vi "校准记录.vi"(8 "error in (no error)":errorcluster, 9 "曲线模型":T1={"标液浓度1"=0.0, "测量吸光度1"=0.0, "样品1启用"=FALSE, "标液浓度2"=0.0, "测量吸光度2"=0.0, "样品2启用"=FALSE, "标液浓度3"=0.0, "测量吸光度3"=0.0, "样品3启用"=FALSE, "标液浓度4"=0.0, "测量吸光度4"=0.0, "样品4启用"=FALSE, "标液浓度5"=0.0, "测量吸光度5"=0.0, "样品5启用"=FALSE, "模型"=enum."线性", "精度"=4.0, "XY图"=[], "拟合公式"="", "r^2"=0.0, "标样一校准时间"=timestamp(0 s since 1904-01-01), "标样二校准时间"=timestamp(0 s since 1904-01-01), "标样三校准时间"=timestamp(0 s since 1904-01-01), "标样四校准时间"=timestamp(0 s since 1904-01-01), "标样五校准时间"=timestamp(0 s since 1904-01-01), "二次方程"={"c"=0.0, "x"=0.0, "x^2"=0.0}, "标定时间"=timestamp(0 s since 1904-01-01), "拟合公式 2"="", "r^2 2"=0.0} {"r^2 2" format="%.7f"; "标定时间" format="%<%m/%d/%y %H:%M:%S>T"; "标样五校准时间" format="%<%m/%d/%y %H:%M:%S>T"; "标样四校准时间" format="%<%m/%d/%y %H:%M:%S>T"; "标样三校准时间" format="%<%m/%d/%y %H:%M:%S>T"; "标样二校准时间" format="%<%m/%d/%y %H:%M:%S>T"; "标样一校准时间" format="%<%m/%d/%y %H:%M:%S>T"; "r^2" format="%.7f"; "测量吸光度5" format="%#.6f"; "测量吸光度4" format="%#.6f"; "测量吸光度3" format="%#.6f"; "测量吸光度2" format="%#.6f"; "测量吸光度1" format="%#.6f"}, 10 "量程":enum16{"低量程", "高量程"}(ring), 11 "校准参数":u16(ring) items=["总氮"=2, "总磷"=1]) -> (0 "error out":errorcluster)   [LabVIEW 2016, in "斯坦道CODMn新电路板.lvlib"]
uses:
  <vilib>/addons/database/Auxilliary.llb/DB Tools Column Info.ctl
  <vilib>/addons/database/Auxilliary.llb/DB Tools DataTypes.ctl
  <vilib>/addons/database/NI_Database_API.lvlib
  <vilib>/Utility/VariantDataType/VariantType.lvlib
panel:
  out "结果字符串":string
  in  "data in":T2
  # "校准时间"
  # "标液浓度"
  # "吸光值显示"
  # "标液一"
  # "标液二"
  # "标液三"
  # "零点"
  # "跨度"
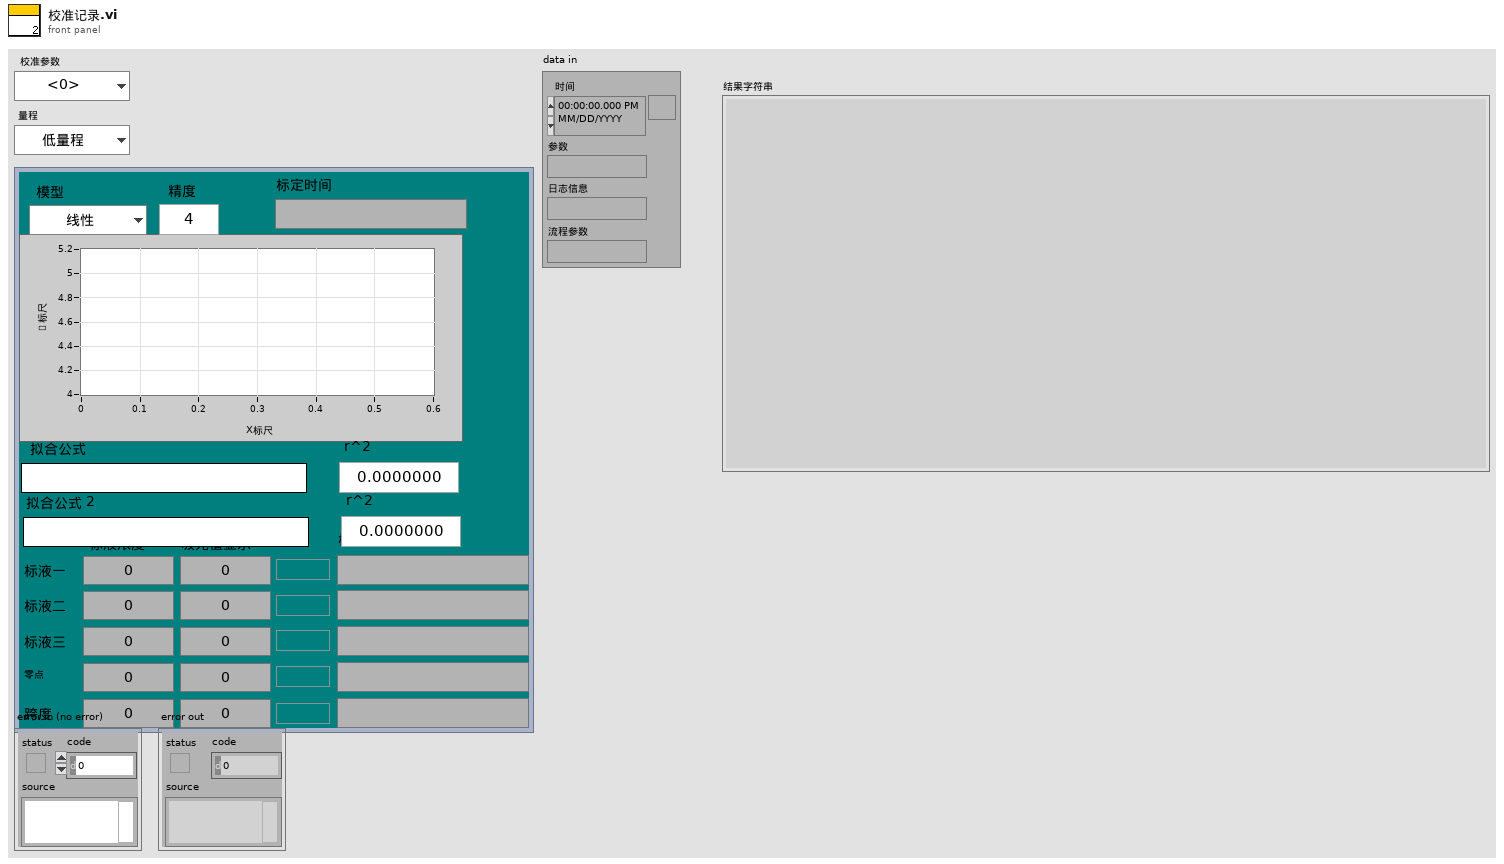
[diagram p1: front panel]
types:
  T1 = cluster{"标液浓度1":dbl, "测量吸光度1":dbl, "样品1启用":bool, "标液浓度2":dbl, "测量吸光度2":dbl, "样品2启用":bool, "标液浓度3":dbl, "测量吸光度3":dbl, "样品3启用":bool, "标液浓度4":dbl, "测量吸光度4":dbl, "样品4启用":bool, "标液浓度5":dbl, "测量吸光度5":dbl, "样品5启用":bool, "模型":enum32{"线性", "多项式", "折线"}, "精度":dbl, "XY图":cluster{"X Values":dbl[], "Y Values":dbl[]}[], "拟合公式":string, "r^2":dbl, "标样一校准时间":timestamp, "标样二校准时间":timestamp, "标样三校准时间":timestamp, "标样四校准时间":timestamp, "标样五校准时间":timestamp, "二次方程":cluster{"c":dbl, "x":dbl, "x^2":dbl}, "标定时间":timestamp, "拟合公式 2":string, "r^2 2":dbl}
  T2 = cluster{"时间":timestamp, "参数":string, "日志信息":string, "流程参数":string}
  T3 = typedef "NI_Database_API.lvlib/DB Tools Column Info.ctl" = cluster{"column name":string, "data type":T4, "size":i32, "allow null?":bool}
  T4 = typedef "NI_Database_API.lvlib/DB Tools DataTypes.ctl" = enum16{"String", "Long (I32)", "Single (SGL)", "Double (DBL)", "Date/Time", "Binary"}
  T5 = typedef "VariantType.lvlib/Type.ctl" = enum8{"Invalid Type", "Void", "I8", "I16", "I32", "I64", "U8", "U16", "U32", "U64", "Single Float", "Double Float", "Extended Float", "Single Complex", "Double Complex", "Extended Complex", "Enum U8", "Enum U16", "Enum U32", "Enum U64", "Single Float With Unit", "Double Float With Unit", "Extended Float With Unit", "Single Complex with Unit", "Double Complex with Unit", "Extended Complex with Unit", "Boolean", "String", "Path", "Picture", "Tag", "Array", "Cluster", "Variant", "LV Variant", "Waveform", "Timestamp", "Digital Waveform", "Digital Data", "ExpressData", "Refnum", "External Data", "VI", "Poly VI", "LabVIEW Class Instance", "Fixed Point"}
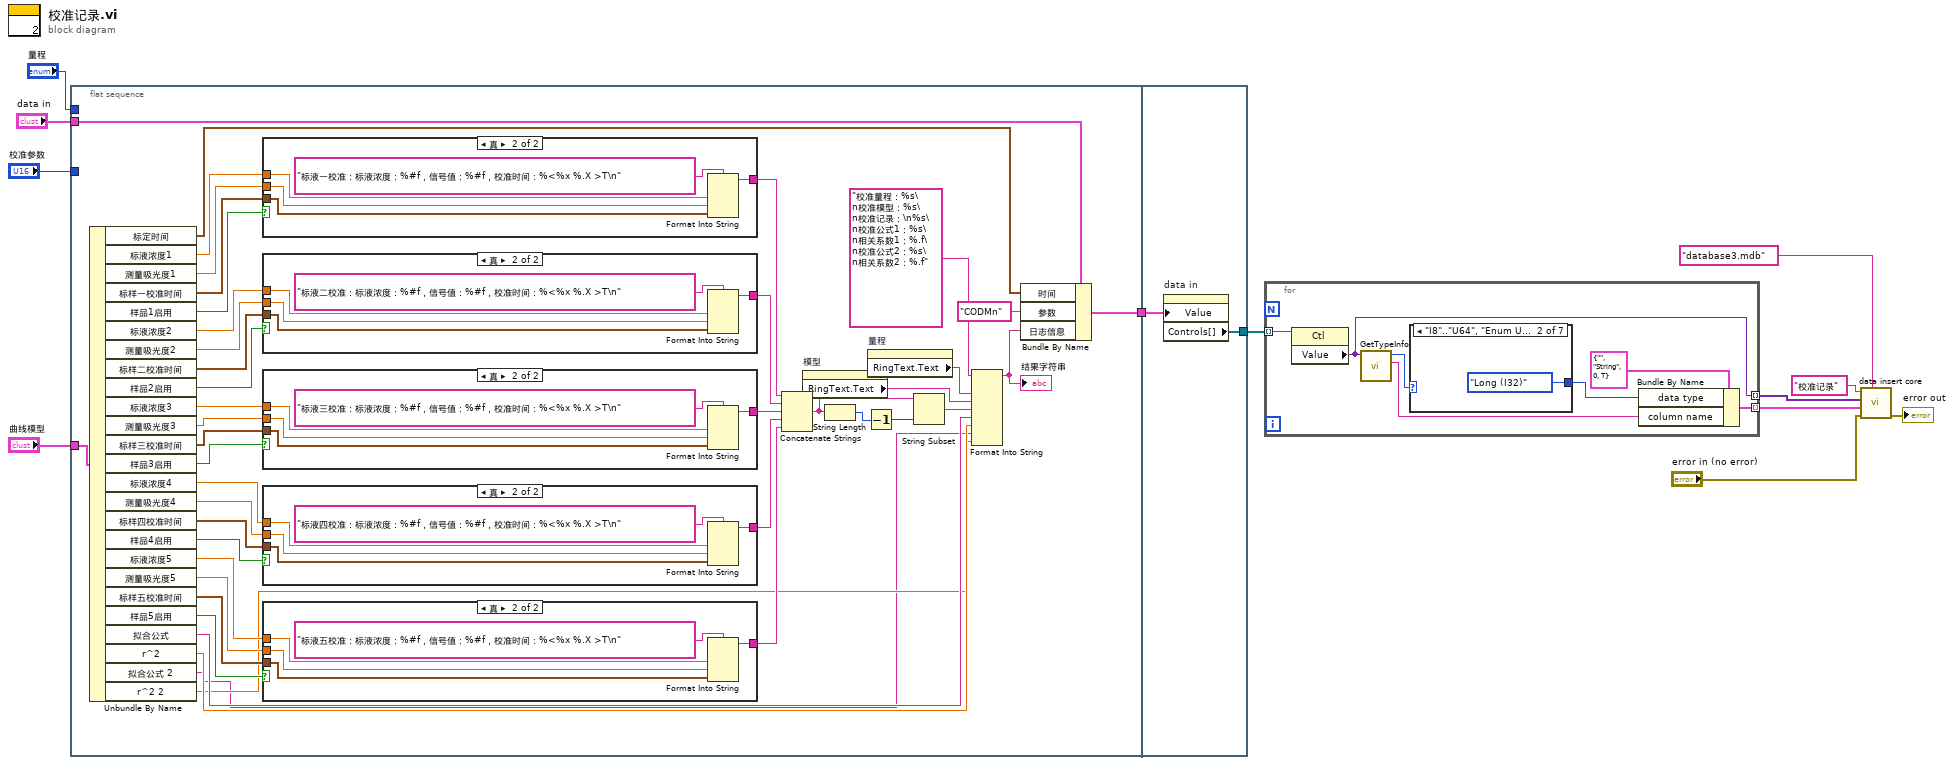
[diagram p0: block diagram]
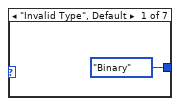
[diagram p7: hidden frame]
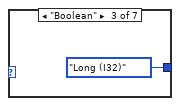
[diagram p8: hidden frame]
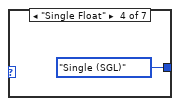
[diagram p9: hidden frame]
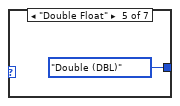
[diagram p10: hidden frame]
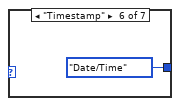
[diagram p11: hidden frame]
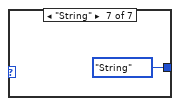
[diagram p12: hidden frame]
diagram:
  n1 = flat-sequence {
    tunnel: "校准参数" -> [_]
    tunnel: "量程" -> [_]
    tunnel: "曲线模型" -> [w50]
    tunnel: "data in" -> [w54]
    tunnel: [w53] -> w2
    tunnel: [w81] -> w11
    tunnel: w2 -> [w80]
    frame #0 {
      n2 = Unbundle By Name(w50) -> ("标定时间"=w18:timestamp, "标液浓度1"=w48:dbl, "测量吸光度1"=w47:dbl, "标样一校准时间"=w46:timestamp, "样品1启用"=w49:bool, "标液浓度2"=w45:dbl, "测量吸光度2"=w44:dbl, "标样二校准时间"=w43:timestamp, "样品2启用"=w42:bool, "标液浓度3"=w41:dbl, "测量吸光度3"=w40:dbl, "标样三校准时间"=w39:timestamp, "样品3启用"=w38:bool, "标液浓度4"=w37:dbl, "测量吸光度4"=w36:dbl, "标样四校准时间"=w35:timestamp, "样品4启用"=w34:bool, "标液浓度5"=w33:dbl, "测量吸光度5"=w32:dbl, "标样五校准时间"=w31:timestamp, "样品5启用"=w30:bool, "拟合公式"=w24:string, "r^2"=w23:dbl, "拟合公式 2"=w16:string, "r^2 2"=w17:dbl)
      n3 = case shown="真" w49 {
        tunnel: w48 -> [_ w78]
        tunnel: w47 -> [_ w77]
        tunnel: w46 -> [_ w76]
        tunnel: [_ w75] -> w29
        frame False {
        }
        frame True {
          n4 = Format Into String(format string="标液一校准：标液浓度：%#f，信号值：%#f，校准时间：%<%x %.X >T\n" ("格式字符串"), w78, w77, w76) -> (resulting string=w75:string)  [unwired: 2 in, 1 out]
        }
      }
      n5 = case shown="真" w42 {
        tunnel: w45 -> [_ w73]
        tunnel: w44 -> [_ w72]
        tunnel: w43 -> [_ w71]
        tunnel: [_ w70] -> w28
        frame False {
        }
        frame True {
          n6 = Format Into String(format string="标液二校准：标液浓度：%#f，信号值：%#f，校准时间：%<%x %.X >T\n" ("格式字符串"), w73, w72, w71) -> (resulting string=w70:string)  [unwired: 2 in, 1 out]
        }
      }
      n7 = case shown="真" w38 {
        tunnel: w41 -> [_ w68]
        tunnel: w40 -> [_ w67]
        tunnel: w39 -> [_ w66]
        tunnel: [_ w65] -> w27
        frame False {
        }
        frame True {
          n8 = Format Into String(format string="标液三校准：标液浓度：%#f，信号值：%#f，校准时间：%<%x %.X >T\n" ("格式字符串"), w68, w67, w66) -> (resulting string=w65:string)  [unwired: 2 in, 1 out]
        }
      }
      n9 = case shown="真" w34 {
        tunnel: w37 -> [_ w63]
        tunnel: w36 -> [_ w62]
        tunnel: w35 -> [_ w61]
        tunnel: [_ w60] -> w26
        frame False {
        }
        frame True {
          n10 = Format Into String(format string="标液四校准：标液浓度：%#f，信号值：%#f，校准时间：%<%x %.X >T\n" ("格式字符串"), w63, w62, w61) -> (resulting string=w60:string)  [unwired: 2 in, 1 out]
        }
      }
      n11 = case shown="真" w30 {
        tunnel: w33 -> [_ w58]
        tunnel: w32 -> [_ w57]
        tunnel: w31 -> [_ w56]
        tunnel: [_ w55] -> w25
        frame False {
        }
        frame True {
          n12 = Format Into String(format string="标液五校准：标液浓度：%#f，信号值：%#f，校准时间：%<%x %.X >T\n" ("格式字符串"), w58, w57, w56) -> (resulting string=w55:string)  [unwired: 2 in, 1 out]
        }
      }
      n13 = Concatenate Strings(w29, w28, w27, w26, w25) -> (w21:string)
      n14 = property on="模型" class="Enum (严格)"() -> ("RingText.Text"=w14:string)  [unwired: 2 in, 2 out]
      n15 = String Length(string=w21) -> (length=w20:i32)
      n16 = Decrement(x=w20) -> (x-1=w19:i32)
      n17 = property on="量程" class="Enum (严格)"() -> ("RingText.Text"=w15:string)  [unwired: 2 in, 2 out]
      n18 = String Subset(string=w21, length (rest)=w19) -> (substring=w22:string)  [unwired: 1 in]
      n19 = Format Into String(format string="校准量程：%s\n校准模型：%s\n校准记录：\n%s\n校准公式1：%s\n相关系数1：%.f\n校准公式2：%s\n相关系数2：%.f" ("格式字符串"), w15, w14, w22, w24, w23, w16, w17) -> (resulting string=w52:string)  [unwired: 2 in, 1 out]
      "结果字符串" <- w52
      n20 = Bundle By Name(cluster=w54, "时间"=w18, "参数"="CODMn", "日志信息"=w52) -> (w53:T2)
    }
    frame #1 {
      n21 = property on="data in" class="Clust (严格)"("Value"=w80) -> ("Controls[]"=w81:refnum<vi>[])  [unwired: 2 in, 2 out]
    }
  }
  n22 = for {
    tunnel: w11 -> [w88] mode=indexing
    tunnel: [w83] -> w9 mode=indexing
    tunnel: [w84] -> w10 mode=indexing
    n23 = property class="Ctl"(reference=w88) -> ("Value"=w83:variant)  [unwired: 1 in, 2 out]
    n24 = call <vilib>:"GetTypeInfo.vi"("Variant"=w83) -> ("Name"=w82:string, "Type Enum"=w86:T5)  [unwired: 6 in, 3 out]
    n25 = case shown="\"I8\"..\"U64\", \"Enum U8\"..\"Enum U64\"" w86 {
      tunnel: [DB_Tools_DataTypes."Binary" ("data type") DB_Tools_DataTypes."Long (I32)" ("data type") DB_Tools_DataTypes."Long (I32)" ("data type") DB_Tools_DataTypes."Single (SGL)" ("data type") DB_Tools_DataTypes."Double (DBL)" ("data type") DB_Tools_DataTypes."Date/Time" ("data type") DB_Tools_DataTypes."String" ("data type")] -> w85
      frame "Invalid Type", Default {
      }
      frame "I8".."U64", "Enum U8".."Enum U64" {
      }
      frame "Boolean" {
      }
      frame "Single Float" {
      }
      frame "Double Float" {
      }
      frame "Timestamp" {
      }
      frame "String" {
      }
    }
    n26 = Bundle By Name(cluster=T3 {"column name"="", "data type"=enum."String", "size"=0, "allow null?"=TRUE} ("column information"), "data type"=w85, "column name"=w82) -> (w84:T3)
  }
  n27 = call "data insert core.vi"("database"="database3.mdb", "error in (no error)"="error in (no error)", "column information"=w10, "data"=w9, "table"="校准记录") -> ("error out"=→"error out":errorcluster)  [unwired: 6 in]
